vi "fromUnicode.vi"(8 "Error In":errorcluster, 10 "string":string, 11 "QTextCodec In":refnum<class "QTextCodec.lvclass">) -> (0 "Error Out":errorcluster, 2 "Value":string, 3 "QTextCodec Out":refnum<class "QTextCodec.lvclass">)   [LabVIEW 2014, in "QTextCodec.lvclass"]
doc: "LabVIEW-specific documentation is not yet available. See <b>https://doc.qt.io/qt-5/qtextcodec.html#fromUnicode</b>"
uses:
  QTextCodec.lvclass
  LQIdentity/LQIdentity.lvclass/LQIdentity.ctl
  LQ Core.lvlib
  LQIdentity/LQIdentity.lvclass
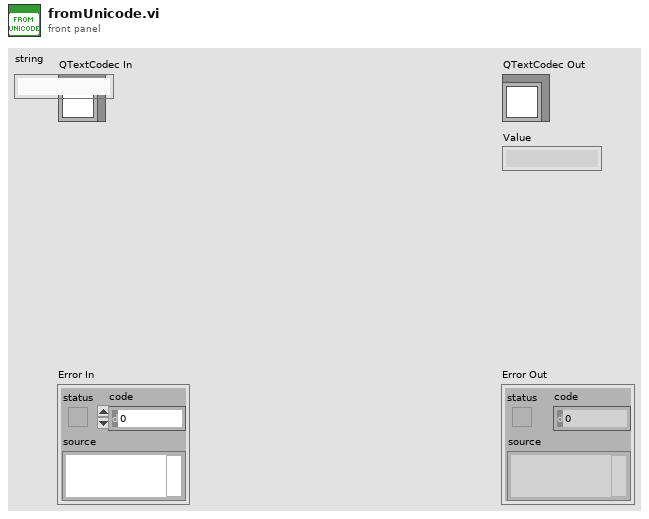
[diagram p1: front panel]
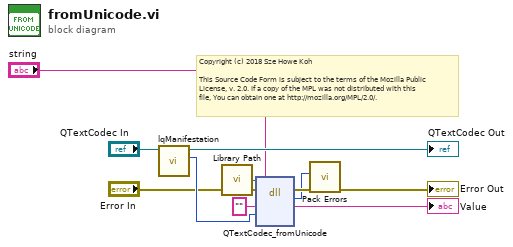
[diagram p0: block diagram]
diagram:
  # "Copyright (c) 2018 Sze Howe Koh\n\nThis Source Code Form is subject to the terms of the Mozilla Public\nLicense, v. 2.0. If a copy of the MPL was not distributed with this\nfile, You can obtain one at http://mozilla.org/MPL/2.0/."
  n1 = call "lqManifestation.vi"("LQIdentity in"="QTextCodec In") -> ("Manifestation"=w6:u64, "LQIdentity out"=→"QTextCodec Out":refnum<class "QTextCodec.lvclass">)  [unwired: 9 in]
  n2 = call "Library Path.vi"() -> ("Library Path"=w7:path)
  n3 = dll-call lib="?" fn="QTextCodec_fromUnicode"(path in=w7, error in="Error In", "_retVal"="" ("retVal"), "_instance"=w6, "string"="string") -> (error out=w4:errorcluster, w2:i32, "_retVal"=→"Value":string)  [unwired: 3 in, 1 out]
  n4 = call "Pack Errors.vi"("Error In"=w4, "Error Code"=w2) -> ("Error Out"=→"Error Out":errorcluster)  [unwired: 9 in]
